vi "Stop.vi"(8 "error in (no error)":errorcluster, 11 "Task in":refnum<class "Channel.lvclass">) -> (0 "error out":errorcluster, 3 "connection ID":i32)   [LabVIEW 2009, in "MicroDAQ.lvlib" / "Channel.lvclass"]
uses:
  <instrlib>/MicroDAQ/Channel/Channel.lvclass
  <instrlib>/MicroDAQ/Channel/Channel.lvclass/Channel.ctl
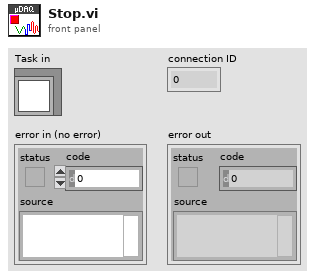
[diagram p1: front panel]
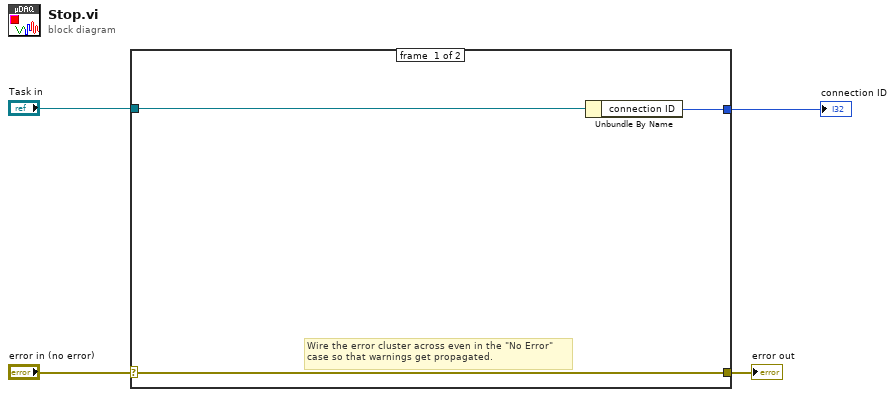
[diagram p0: block diagram]
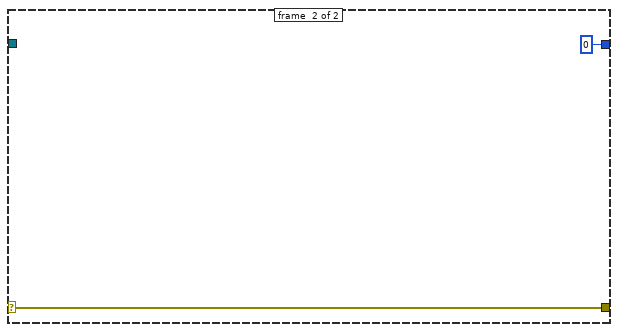
[diagram p2: hidden frame]
diagram:
  n1 = case shown="No Error" "error in (no error)" {
    selector: "error in (no error)" -> [w7 w9]
    tunnel: [w7 w9] -> w3
    tunnel: "Task in" -> [w6 _]
    tunnel: [w5 0 ("connection ID")] -> w1
    frame #0 {
      # "Wire the error cluster across even in the \"No Error\"\ncase so that warnings get propagated."
      n2 = Unbundle By Name(w6) -> ("connection ID"=w5:i32)
    }
    frame #1 {
    }
  }
  "error out" <- w3
  "connection ID" <- w1
